vi "CODCr外部API.vi"() -> ()   [LabVIEW 2016, in "CODCr库.lvlib"]
uses:
  <vilib>/Plasmionique/MB Master/MB_Master/MB_Master.lvclass
panel:
  in  "MB session in":refnum<class "MB_Master.lvclass">
  in  "CODCr外围API":T1
  in  "自动切换量程":bool=TRUE
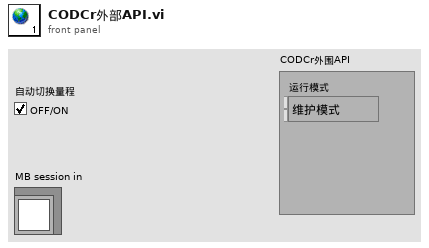
[diagram p1: front panel]
types:
  T1 = cluster{"运行模式":enum16{"维护模式", "常规模式", "应急模式", "质控模式"}}
diagram:
